vi "Create Arbitrary Waveform.vi"(8 "error in (no error)":errorcluster, 10 "Arbitrary Waveform Data":dbl[](array[numeric]), 11 "VISA resource name":refnum<visa-resource-name>) -> (0 "error out":errorcluster, 3 "VISA resource name out":refnum<visa-resource-name>)   [LabVIEW 2016, in "Tektronix AFG 1000 Series.lvlib"]
doc: "Creates an arbitrary waveform in edit memory."
uses:
  Tektronix AFG 1000 Series.lvlib
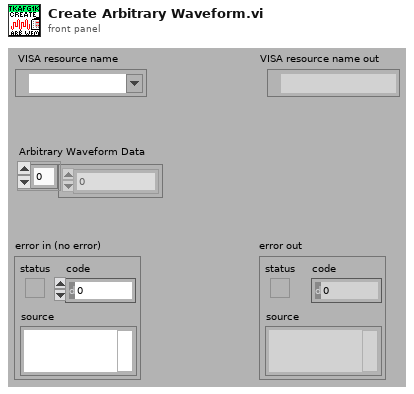
[diagram p1: front panel]
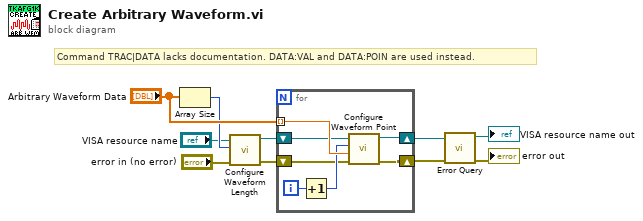
[diagram p0: block diagram]
diagram:
  # "Command TRAC|DATA lacks documentation. DATA:VAL and DATA:POIN are used instead."
  n1 = Array Size(array="Arbitrary Waveform Data") -> (size(s)=w7:i32)
  n2 = call "Configure Waveform Length.vi"("error in (no error)"="error in (no error)", "Set Points (1000)"=w7, "VISA resource name"="VISA resource name") -> ("error out"=w4:errorcluster, "VISA resource name out"=w2:refnum<visa-resource-name>)  [unwired: 7 in]
  n3 = for {
    tunnel: "Arbitrary Waveform Data" -> [w17] mode=indexing
    shift-right: [w11] -> w1
    shift-left: w2 -> [w12]
    shift-right: [w13] -> w3
    shift-left: w4 -> [w14]
    i -> [w15]
    n4 = Increment(x=w15) -> (x+1=w16:i32)
    n5 = call "Configure Waveform Point.vi"("error in (no error)"=w14, "Value (1)"=w17, "Index (1)"=w16, "VISA resource name"=w12) -> ("error out"=w13:errorcluster, "VISA resource name out"=w11:refnum<visa-resource-name>)  [unwired: 6 in]
  }
  n6 = call "Error Query.vi"("error in (no error)"=w3, "VISA resource name"=w1) -> ("error out"=→"error out":errorcluster, "VISA resource name out"=→"VISA resource name out":refnum<visa-resource-name>)  [unwired: 6 in, 2 out]
